vi "MDS.vi"(8 "error in":errorcluster) -> (0 "error out":errorcluster, 3 "out":refnum<class "MDS.lvclass">)   [LabVIEW 2020]
doc: "Multidimensional scaling.\n\n Read more in the :ref:`User Guide <multidimensional_scaling>`.\n\n Parameters\n ----------\n n_components : int, default=2\n Number of dimensions in which to immerse the dissimilarities.\n\n metric : bool, default=True\n If ``True``, perform metric MDS; otherwise, perform nonmetric MDS.\n\n n_init : int, default=4\n Number of times the SMACOF algorithm will be run with different\n initializations. The final results will be the best output of the runs,\n determined by the run with the smallest final stress.\n\n max_iter : int, default=300\n Maximum number of iterations of the SMACOF algorithm for a single run.\n\n verbose : int, default=0\n Level of verbosity.\n\n eps : float, default=1e-3\n Relative tolerance with respect to stress at which to declare\n convergence.\n\n n_jobs : int, default=None\n The number of jobs to use for the computation. If multiple\n initializations are used (``n_init``), each run of the algorithm is\n computed in parallel.\n\n ``None`` means 1 unless in a :obj:`joblib.parallel_backend` context.\n ``-1`` means using all processors. See :term:`Glossary <n_jobs>`\n for more details.\n\n random_state : int, RandomState instance or None, default=None\n Determines the random number generator used to initialize the centers.\n Pass an int for reproducible results across multiple function calls.\n See :term: `Glossary <random_state>`.\n\n dissimilarity : {'euclidean', 'precomputed'}, default='euclidean'\n Dissimilarity measure to use:\n\n - 'euclidean':\n Pairwise Euclidean distances between points in the dataset.\n\n - 'precomputed':\n Pre-computed dissimilarities are passed directly to ``fit`` and\n ``fit_transform``.\n\n Attributes\n ----------\n embedding_ : ndarray of shape (n_samples, n_components)\n Stores the position of the dataset in the embedding space.\n\n stress_ : float\n The final value of the stress (sum of squared distance of the\n disparities and the distances for all constrained points).\n\n dissimilarity_matrix_ : ndarray of shape (n_samples, n_samples)\n Pairwise dissimilarities between the points. Symmetric matrix that:\n\n - either uses a custom dissimilarity matrix by setting `dissimilarity`\n to 'precomputed';\n - or constructs a dissimilarity matrix from data using\n Euclidean distances.\n\n n_iter_ : int\n The number of iterations corresponding to the best stress.\n\n \nAvailable methods:\nFit\nFit Transform\nGet Attributes\nGet Params\nSet Params"
uses:
  MDS.lvclass
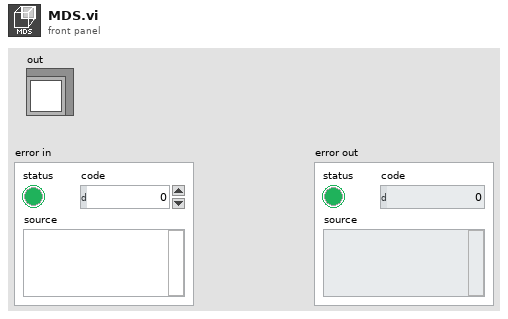
[diagram p1: front panel]
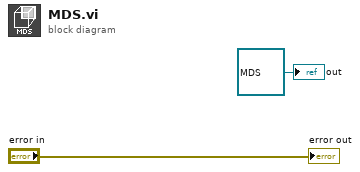
[diagram p0: block diagram]
diagram:
  "out" <- refnum<class "MDS.lvclass"> refnum ("model")
  "error out" <- "error in"
